vi "Aver merged.vi"(8 "error in (no error)":errorcluster, 11 "Control-Client in":refnum<class "Control-Client.lvclass">) -> (0 "error out":errorcluster, 3 "Control-Client out":refnum<class "Control-Client.lvclass">)   [LabVIEW 2019, in "Control-Client.lvclass"]
uses:
  Control-Client.lvclass
  Experiments/Experiment_merged/Experiment_merged.lvclass
  C:/Users/elysium/Documents/dev/TRANCON/Classes/Experiments/Experiment.lvclass
  Control-Client.lvclass/Control-Client.ctl
  Experiments/Experiment.lvclass
panel:
  out "Data aver":dbl[][](array[numeric])
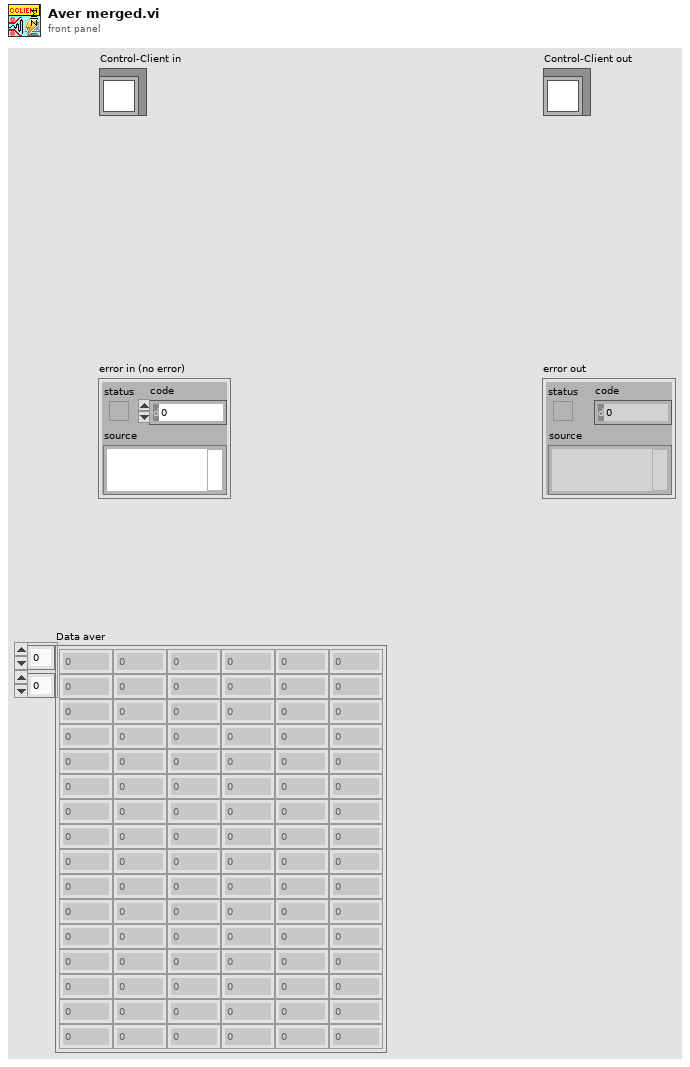
[diagram p1: front panel]
types:
  T1 = cluster{"Max Y pixel":i32, "Min Y pixel":i32, "Max X pixel":i32, "Min X pixel":i32}
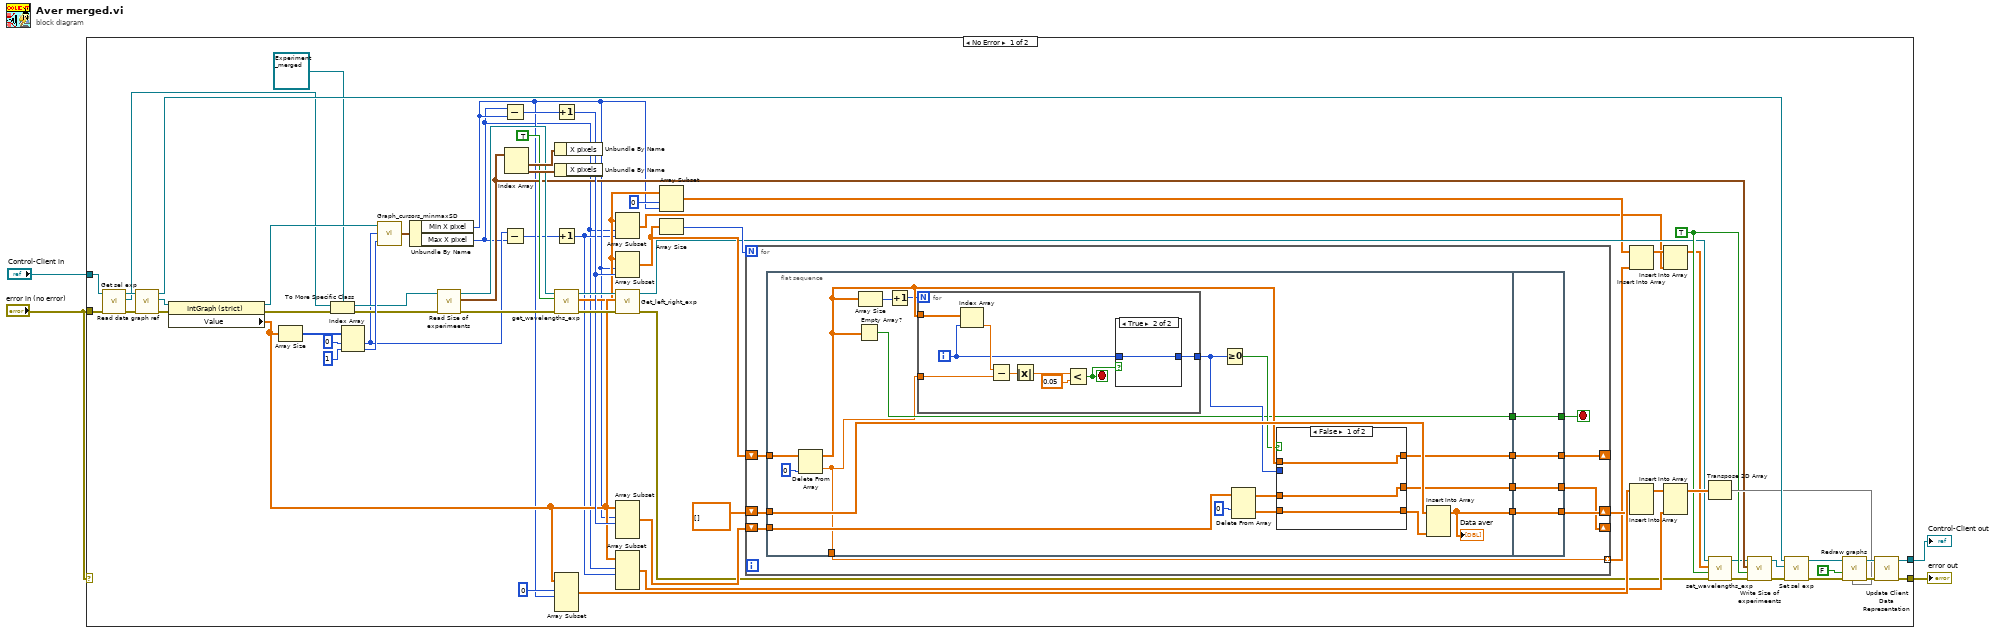
[diagram p0: block diagram]
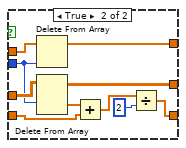
[diagram p2: hidden frame]
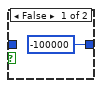
[diagram p3: hidden frame]
diagram:
  n1 = case shown="No Error" "error in (no error)" {
    selector: "error in (no error)" -> [_ w130]
    tunnel: [w70 w130] -> w4
    tunnel: [w69 w129] -> w2
    tunnel: "Control-Client in" -> [w68 w129]
    tunnel: "error in (no error)" -> [w67 _]
    frame No Error {
      w19 = TRUE ("Temp")
      n2 = call "Get sel exp.vi"("error in (no error)"=w67, "Control-Client in"=w68) -> ("error out"=w65:errorcluster, "Sel experiment"=w42:refnum<class "Experiment.lvclass">, "Control-Client out"=w66:refnum<class "Control-Client.lvclass">)  [unwired: 7 in]
      n3 = call "Read data graph ref.vi"("error in (no error)"=w65, "Control-Client in"=w66) -> ("error out"=w63:errorcluster, "Exp data graph ref"=w64:refnum<vi>, "Control-Client out"=w60:refnum<class "Control-Client.lvclass">)  [unwired: 7 in]
      n4 = property class="IntGraph (strict)"(reference=w64, error in=w63) -> (reference out=w59:refnum<vi>, error out=w43:errorcluster, "Value"=w29:dbl[][])
      n5 = Array Size(array=w29) -> (size(s)=w58:i32[])
      n6 = To More Specific Class(target class=refnum<class "Experiment_merged.lvclass"> refnum ("Experiment_merged in"), reference=w42, error in=w43) -> (specific class reference=w47:refnum<class "Experiment_merged.lvclass">, error out=w46:errorcluster)
      n7 = Index Array(array=w58, index #1=0 ("index"), index #2=1 ("index")) -> (element #1=w8:i32, element #2=w57:i32)
      n8 = call "Graph_cursors_minmaxSD.vi"("Max Y pixel"=w57, "Max X pixel"=w8, "GRAPH EXPERIMENTAL DATA"=w59) -> ("max/min XY pixels"=w56:T1)
      n9 = Unbundle By Name(w56) -> ("Min X pixel"=w9:i32, "Max X pixel"=w5:i32)
      n10 = call-dynamic "Read Size of experimeents.vi"("error in (no error)"=w46, "Experiment_merged in"=w47) -> ("error out"=w40:errorcluster, "Size of experimeents"=w22:cluster{"X pixels":i32, "Y pixels":i32}[], "Experiment_merged out"=w39:refnum<class "Experiment_merged.lvclass">)  [unwired: 7 in]
      n11 = Subtract(x=w5, y=w9) -> (x-y=w55:i32)
      n12 = Subtract(x=w8, y=w5) -> (x-y=w7:i32)
      n13 = Index Array(array=w22) -> (element #1=w45:cluster{"X pixels":i32, "Y pixels":i32}, element #2=w44:cluster{"X pixels":i32, "Y pixels":i32})  [unwired: 2 in]
      n14 = Increment(x=w55) -> (x+1=w31:i32)
      n15 = Unbundle By Name(w45) -> ()  [unwired: 1 out]
      n16 = Unbundle By Name(w44) -> ()  [unwired: 1 out]
      n17 = Increment(x=w7) -> (x+1=w6:i32)
      n18 = call "get_wavelengths_exp.vi"("error in (no error)"=w40, "Temp"=TRUE, "Experiment.lvclass in"=w39) -> ("error out"=w37:errorcluster, "wavelengths"=w11:dbl[], "Experiment.lvclass out"=w36:refnum<class "Experiment_merged.lvclass">)  [unwired: 6 in]
      n19 = Array Subset(array=w29, index (row)=0 ("index"), length (row)=w9) -> (w28:dbl[][])  [unwired: 2 in]
      n20 = Array Subset(array=w11, index=w5, length=w6) -> (w13:dbl[])
      n21 = Array Subset(array=w11, index=w9, length=w31) -> (w33:dbl[])
      n22 = call "Get_left_right_exp.vi"("error in (no error)"=w37, "Data"=w29, "Experiment_merged in"=w36) -> ("error out"=w21:errorcluster, "Experiment_merged out"=w18:refnum<class "Experiment_merged.lvclass">)  [unwired: 5 in, 2 out]
      n23 = Array Subset(array=w29, index (row)=w9, length (row)=w31) -> (w32:dbl[][])  [unwired: 2 in]
      n24 = Array Subset(array=w29, index (row)=w5, length (row)=w6) -> (w25:dbl[][])  [unwired: 2 in]
      n25 = Array Subset(array=w11, index=0, length=w9) -> (w16:dbl[])
      n26 = Array Size(array=w33) -> (size(s)=w35:i32)
      n27 = for {
        N: w35 -> [_]
        shift-right: [w80] -> _
        shift-left: w33 -> [w82]
        shift-right: [w79] -> w27
        shift-left: dbl[][] [] ("Data aver") -> [w81]
        shift-right: [w78] -> _
        shift-left: w32 -> [w77]
        tunnel: [w71] -> w15 mode=indexing
        stop <- w72 stop-if-true
        n28 = flat-sequence {
          tunnel: w82 -> [w100]
          tunnel: w81 -> [w99]
          tunnel: w77 -> [w89]
          tunnel: [w96] -> w76
          tunnel: [w95] -> w75
          tunnel: [w90] -> w74
          tunnel: [w85] -> w73
          tunnel: [w83] -> w71
          tunnel: [w126] -> w78
          tunnel: [w127] -> w79
          tunnel: [w128] -> w80
          tunnel: w76 -> [w128]
          tunnel: w75 -> [w127]
          tunnel: w74 -> [w126]
          tunnel: w73 -> [w125]
          tunnel: [w125] -> w72
          frame #0 {
            n29 = Delete From Array(array=w100, index=0) -> (deleted portion=w83:dbl, array with subset deleted=w94:dbl[])  [unwired: 1 in]
            n30 = Empty Array?(array=w94) -> (empty?=w85:bool)
            n31 = Array Size(array=w94) -> (size(s)=w93:i32)
            n32 = Increment(x=w93) -> (x+1=w84:i32)
            n33 = for {
              N: w84 -> [_]
              tunnel: w83 -> [w119]
              tunnel: w94 -> [w122]
              tunnel: [w121] -> w91
              i -> [w114]
              stop <- w115 stop-if-true
              n34 = Index Array(array=w122, index=w114) -> (element=w120:dbl)
              n35 = Subtract(x=w120, y=w119) -> (x-y=w118:dbl)
              n36 = Absolute Value(x=w118) -> (abs(x)=w117:dbl)
              n37 = Less?(x=w117, y=0.05) -> (x < y?=w115:bool)
              n38 = case shown="True" w115 {
                tunnel: w114 -> [_ w124]
                tunnel: [-100000 w124] -> w121
                frame False {
                }
                frame True {
                }
              }
            }
            n39 = Greater Or Equal To 0?(x=w91) -> (x >= 0?=w92:bool)
            n40 = Delete From Array(array=w89, index (row)=0) -> (deleted portion=w87:dbl[], array with subset deleted=w88:dbl[][])  [unwired: 2 in]
            n41 = case shown="False" w92 {
              tunnel: w88 -> [w102 w107]
              tunnel: [w101 w111] -> w98
              tunnel: w94 -> [w103 w110]
              tunnel: w91 -> [_ w104]
              tunnel: [w103 w109] -> w96
              tunnel: [w102 w105] -> w90
              tunnel: w87 -> [w101 w108]
              frame False {
              }
              frame True {
                n42 = Delete From Array(array=w110, index=w104) -> (array with subset deleted=w109:dbl[])  [unwired: 1 in, 1 out]
                n43 = Delete From Array(array=w107, index (row)=w104) -> (deleted portion=w106:dbl[], array with subset deleted=w105:dbl[][])  [unwired: 2 in]
                n44 = Add(x=w106, y=w108) -> (x+y=w113:dbl[])
                n45 = Divide(x=w113, y=2 ("Numeric")) -> (x/y=w111:dbl[])
              }
            }
            n46 = Insert Into Array(array=w99, new element=w98) -> (w95:dbl[][])  [unwired: 2 in]
            "Data aver" <- w95
          }
          frame #1 {
          }
        }
      }
      n47 = Insert Into Array(array=w16, new element=w15) -> (w14:dbl[])  [unwired: 1 in]
      n48 = Insert Into Array(array=w28, new element=w27) -> (w26:dbl[][])  [unwired: 2 in]
      n49 = Insert Into Array(array=w14, new element=w13) -> (w12:dbl[])  [unwired: 1 in]
      n50 = Insert Into Array(array=w26, new element=w25) -> (w24:dbl[][])  [unwired: 2 in]
      n51 = Transpose 2D Array(2D array=w24) -> (transposed array=w23:dbl[][])
      n52 = call "set_wavelengths_exp.vi"("error in (no error)"=w21, "Temp"=w19, "wavelengths"=w12, "Experiment.lvclass in"=w18) -> ("error out"=w20:errorcluster, "Experiment.lvclass out"=w17:refnum<class "Experiment_merged.lvclass">)  [unwired: 6 in]
      n53 = call-dynamic "Write Size of experimeents.vi"("error in (no error)"=w20, "Temp"=w19, "Size of experimeents"=w22, "Experiment_merged in"=w17) -> ("error out"=w48:errorcluster, "Experiment_merged out"=w49:refnum<class "Experiment_merged.lvclass">)  [unwired: 6 in]
      n54 = call "Set sel exp.vi"("error in (no error)"=w48, "Experiment"=w49, "Control-Client in"=w60) -> ("error out"=w52:errorcluster, "Control-Client out"=w54:refnum<class "Control-Client.lvclass">)  [unwired: 7 in]
      n55 = call "Redraw graphs.vi"("Data"=w23, "error in (no error)"=w52, "Selected exp"=FALSE, "Control-Client in"=w54) -> ("error out"=w51:errorcluster, "Control-Client out"=w53:refnum<class "Control-Client.lvclass">)  [unwired: 6 in]
      n56 = call "Update Client Data Representation.vi"("error in (no error)"=w51, "Control-Client in"=w53) -> ("error out"=w70:errorcluster, "Control-Client out"=w69:refnum<class "Control-Client.lvclass">)  [unwired: 8 in]
    }
    frame Error {
    }
  }
  "error out" <- w4
  "Control-Client out" <- w2
